vi "Do[Core].vi"(0 "ControlAction in":refnum<class "DoValueSignal.lvclass">, 5 "Ctl Refnum in":refnum<vi>, 11 "error in (no error)":errorcluster) -> (4 "ControlAction out":refnum<class "DoValueSignal.lvclass">, 6 "Ctl Refnum out":refnum<vi>, 15 "error out":errorcluster)   [LabVIEW 2016, in "DoValueSignal.lvclass"]
uses:
  DoValueSignal.lvclass
  VIActionBase/ControlActionBase.lvclass
panel:
  in  "OK":bool
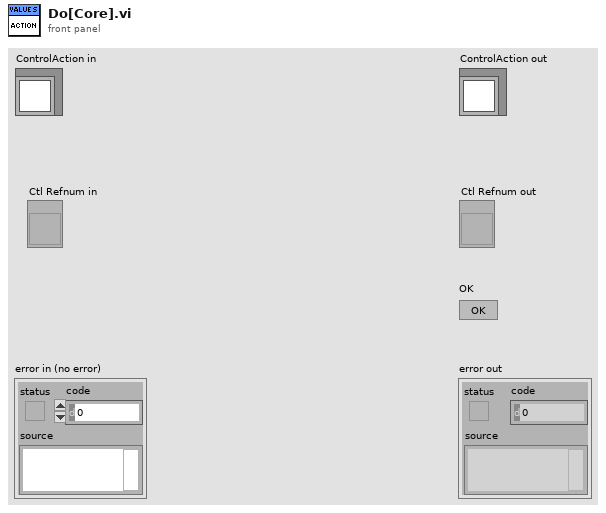
[diagram p1: front panel]
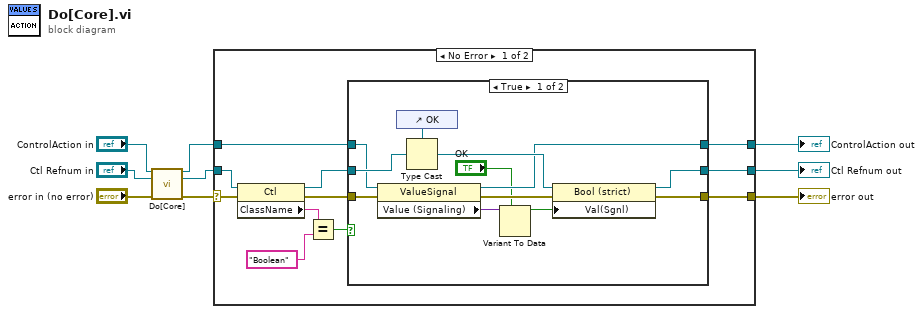
[diagram p0: block diagram]
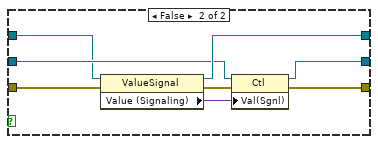
[diagram p2: hidden frame]
diagram:
  n1 = call-parent "Do[Core].vi"("ControlAction in"="ControlAction in", "Ctl Refnum in"="Ctl Refnum in", "error in (no error)"="error in (no error)") -> ("ControlAction out"=w3:refnum<class "DoValueSignal.lvclass">, "Ctl Refnum out"=w2:refnum<vi>, "error out"=w5:errorcluster)  [unwired: 10 in]
  n2 = case shown="No Error" w5 {
    selector: w5 -> [w14 w43]
    tunnel: [w20 w43] -> w9
    tunnel: [w19 w42] -> w8
    tunnel: [w18 w41] -> w7
    tunnel: w2 -> [w16 w42]
    tunnel: w3 -> [w17 w41]
    frame No Error {
      n3 = property class="Ctl"(reference=w16, error in=w14) -> (reference out=w15:refnum<vi>, error out=w13:errorcluster, "ClassName"=w12:string)
      n4 = Equal?(x=w12, y="Boolean") -> (x = y?=w10:bool)
      n5 = case shown="True" w10 {
        tunnel: [w25 w40] -> w20
        tunnel: [w27 w39] -> w19
        tunnel: [w28 w38] -> w18
        tunnel: w13 -> [w24 w37]
        tunnel: w15 -> [w32 w36]
        tunnel: w17 -> [w29 w34]
        frame True {
          n6 = property class="ValueSignal"(reference=w29, error in=w24) -> (reference out=w28:refnum<class "DoValueSignal.lvclass">, error out=w23:errorcluster, "Value (Signaling)"=w26:variant)
          n7 = control-ref of="OK"() -> (w31:refnum<vi>)
          n8 = Type Cast(type=w31, x=w32) -> (*(type *) &x=w30:refnum<vi>)
          n9 = Variant To Data(type="OK", Variant=w26) -> (data=w21:bool)  [unwired: 1 in, 1 out]
          n10 = property class="Bool (strict)"(reference=w30, error in=w23, "Val(Sgnl)"=w21) -> (reference out=w27:refnum<vi>, error out=w25:errorcluster)
        }
        frame False {
          n11 = property class="ValueSignal"(reference=w34, error in=w37) -> (reference out=w38:refnum<class "DoValueSignal.lvclass">, error out=w35:errorcluster, "Value (Signaling)"=w33:variant)
          n12 = property class="Ctl"(reference=w36, error in=w35, "Val(Sgnl)"=w33) -> (reference out=w39:refnum<vi>, error out=w40:errorcluster)
        }
      }
    }
    frame Error {
    }
  }
  "error out" <- w9
  "ControlAction out" <- w7
  "Ctl Refnum out" <- w8
